vi "5302GetTC.vi"(8 "error in (no error)":errorcluster, 11 "VISA Resource Name":refnum<visa-resource-name>) -> (0 "error out":errorcluster, 1 "data string":string, 2 "Time Constant":dbl format="%.4e", 3 "VISA Resource Name Out":refnum<visa-resource-name>)   [LabVIEW 2015]
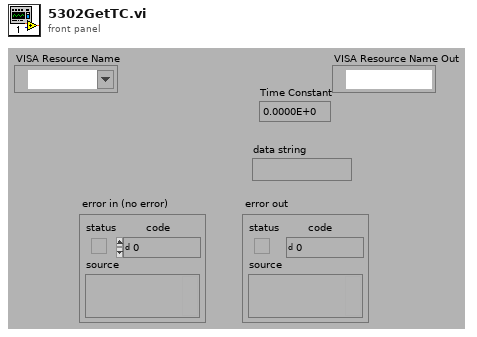
[diagram p1: front panel]
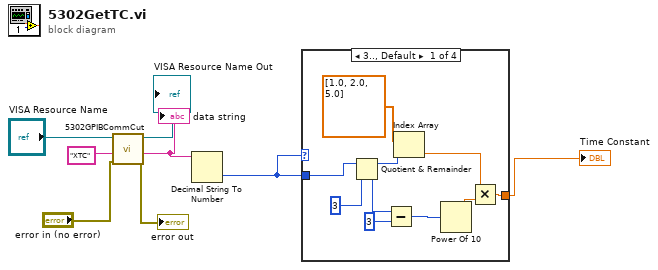
[diagram p0: block diagram]
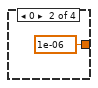
[diagram p2: hidden frame]
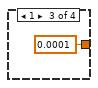
[diagram p3: hidden frame]
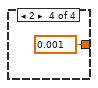
[diagram p4: hidden frame]
diagram:
  n1 = call "5302GPIBCommCut.vi"("error in (no error)"="error in (no error)", "data string in"="XTC" ("data string"), "VISA Resource Name"="VISA Resource Name") -> ("error out"=→"error out":errorcluster, "data string out"=w4:string, "VISA Resource Name Out"=→"VISA Resource Name Out":refnum<visa-resource-name>)  [unwired: 2 in, 4 out]
  "data string" <- w4
  n2 = Decimal String To Number(string=w4) -> (number=w3:i32)  [unwired: 1 in, 2 out]
  n3 = case shown="3.., Default" w3 {
    tunnel: [w16 1e-06 0.0001 0.001] -> w5
    tunnel: w3 -> [w15 _ _ _]
    frame 3.., Default {
      n4 = Quotient & Remainder(x=w15, y=3) -> (x-y*floor(x/y)=w11:i32, floor(x/y)=w13:i32)
      n5 = Subtract(x=w13, y=3) -> (x-y=w14:i32)
      n6 = Index Array(array=dbl[] [1.0, 2.0, 5.0] ("Input Array"), index=w11) -> (element=w9:dbl)
      n7 = Power Of 10(x=w14) -> (10^x=w17:dbl)
      n8 = Multiply(x=w9, y=w17) -> (x*y=w16:dbl)
    }
    frame 0 {
    }
    frame 1 {
    }
    frame 2 {
    }
  }
  "Time Constant" <- w5
